vi "HB_SetTime.vi"(8 "error in (no error)":errorcluster, 10 "Time Stamp":timestamp, 11 "HBDeviceRef":T1) -> (0 "error IO":errorcluster, 3 "HBDeviceRef":T1)   [LabVIEW 2016]
uses:
  <vilib>/Rock Robotics/WPI/SerialPort/WPI_SerialPortRef.ctl
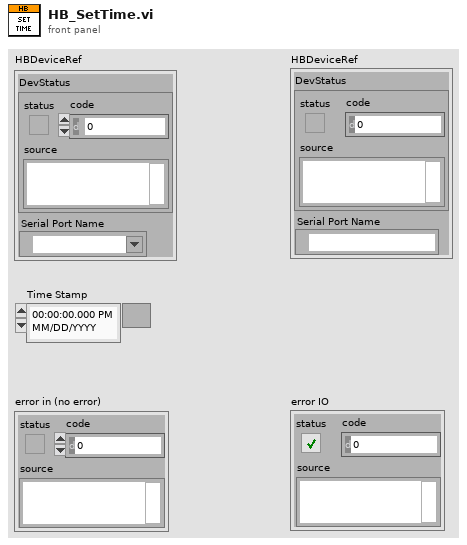
[diagram p1: front panel]
types:
  T1 = typedef "WPI_SerialPortRef.ctl" = cluster{"DevStatus":errorcluster, "Serial Port Name":refnum<visa-resource-name>}
  T2 = typedef "LVDateTimeRec.ctl" = cluster{"fractional second":dbl, "second":i32, "minute":i32, "hour":i32, "day of month":i32, "month":i32, "year":i32, "day of week":i32, "day of year":i32, "DST":i32}
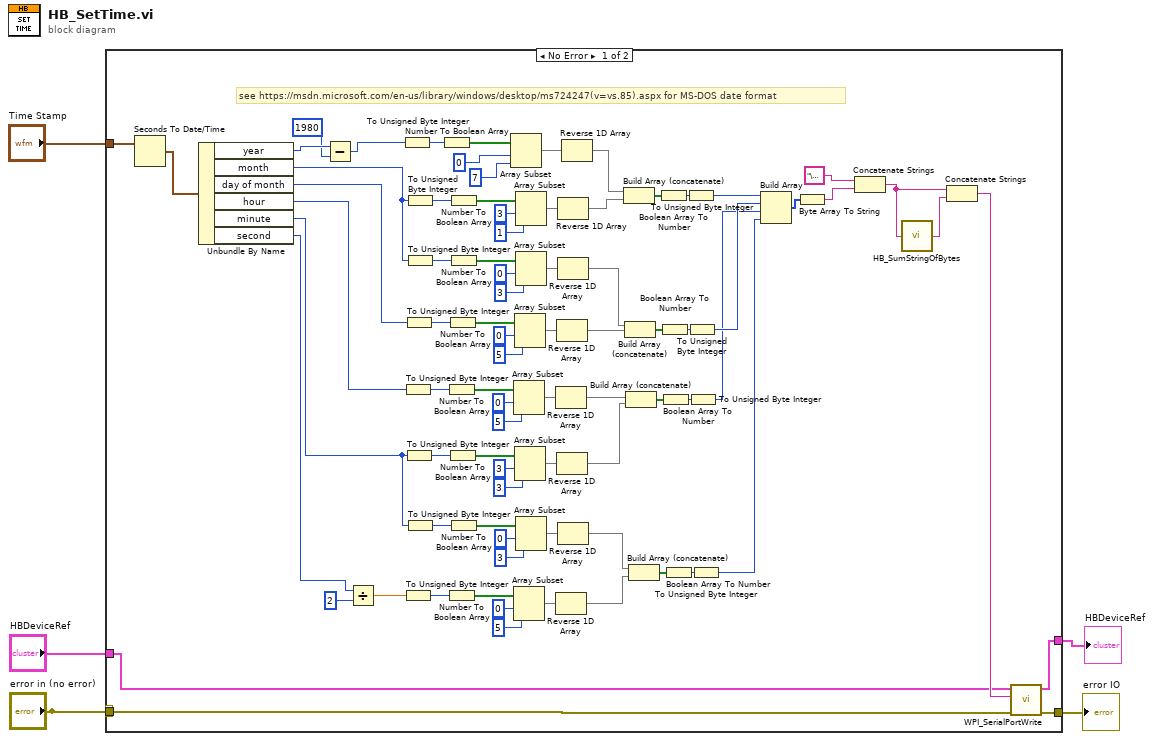
[diagram p0: block diagram]
diagram:
  n1 = case shown="No Error" "error in (no error)" {
    selector: "error in (no error)" -> [w9 w88]
    tunnel: "HBDeviceRef" -> [w6 w89]
    tunnel: "error in (no error)" -> [_ _]
    tunnel: [w7 w89] -> w2
    tunnel: [w8 w88] -> w3
    tunnel: "Time Stamp" -> [w66 _]
    frame No Error {
      # "see https://msdn.microsoft.com/en-us/library/windows/desktop/ms724247(v=vs.85).aspx for MS-DOS date format"
      n2 = Seconds To Date/Time(time stamp (now)=w66) -> (date time rec=w65:T2)  [unwired: 1 in]
      n3 = Unbundle By Name(w65) -> ("year"=w64:i32, "month"=w12:i32, "day of month"=w41:i32, "hour"=w40:i32, "minute"=w13:i32, "second"=w39:i32)
      n4 = Subtract(x=w64, y=1980) -> (x-y=w62:i32)
      n5 = Divide(x=w39, y=2) -> (x/y=w38:dbl)
      n6 = To Unsigned Byte Integer(number=w62) -> (unsigned 8bit integer=w78:u8)
      n7 = To Unsigned Byte Integer(number=w40) -> (unsigned 8bit integer=w56:u8)
      n8 = To Unsigned Byte Integer(number=w38) -> (unsigned 8bit integer=w46:u8)
      n9 = To Unsigned Byte Integer(number=w41) -> (unsigned 8bit integer=w61:u8)
      n10 = To Unsigned Byte Integer(number=w13) -> (unsigned 8bit integer=w51:u8)
      n11 = To Unsigned Byte Integer(number=w12) -> (unsigned 8bit integer=w83:u8)
      n12 = To Unsigned Byte Integer(number=w12) -> (unsigned 8bit integer=w30:u8)
      n13 = To Unsigned Byte Integer(number=w13) -> (unsigned 8bit integer=w21:u8)
      n14 = Number To Boolean Array(number=w78) -> (Boolean array=w77:bool[])
      n15 = Number To Boolean Array(number=w56) -> (Boolean array=w52:bool[])
      n16 = Number To Boolean Array(number=w46) -> (Boolean array=w42:bool[])
      n17 = Number To Boolean Array(number=w61) -> (Boolean array=w57:bool[])
      n18 = Number To Boolean Array(number=w51) -> (Boolean array=w47:bool[])
      n19 = Number To Boolean Array(number=w83) -> (Boolean array=w79:bool[])
      n20 = Number To Boolean Array(number=w30) -> (Boolean array=w26:bool[])
      n21 = Number To Boolean Array(number=w21) -> (Boolean array=w17:bool[])
      n22 = Array Subset(array=w77, index=0, length=7) -> (w68:bool[])
      n23 = Array Subset(array=w52, index=0, length=5) -> (w53:bool[])
      n24 = Array Subset(array=w42, index=0, length=5) -> (w43:bool[])
      n25 = Array Subset(array=w57, index=0, length=5) -> (w58:bool[])
      n26 = Array Subset(array=w47, index=3, length=3) -> (w48:bool[])
      n27 = Array Subset(array=w79, index=3, length=1) -> (w80:bool[])
      n28 = Array Subset(array=w26, index=0, length=3) -> (w27:bool[])
      n29 = Array Subset(array=w17, index=0, length=3) -> (w18:bool[])
      n30 = Reverse 1D Array(array=w53) -> (reversed array=w22:bool[])
      n31 = Reverse 1D Array(array=w43) -> (reversed array=w14:bool[])
      n32 = Reverse 1D Array(array=w58) -> (reversed array=w24:bool[])
      n33 = Reverse 1D Array(array=w48) -> (reversed array=w16:bool[])
      n34 = Reverse 1D Array(array=w80) -> (reversed array=w72:bool[])
      n35 = Reverse 1D Array(array=w27) -> (reversed array=w25:bool[])
      n36 = Reverse 1D Array(array=w18) -> (reversed array=w15:bool[])
      n37 = Reverse 1D Array(array=w68) -> (reversed array=w67:bool[])
      n38 = Build Array (concatenate)(w67, w72) -> (w71:bool[])
      n39 = Build Array (concatenate)(w25, w24) -> (w35:bool[])
      n40 = Build Array (concatenate)(w22, w16) -> (w33:bool[])
      n41 = Build Array (concatenate)(w15, w14) -> (w31:bool[])
      n42 = Boolean Array To Number(Boolean array=w71) -> (number=w75:u32)
      n43 = Boolean Array To Number(Boolean array=w35) -> (number=w36:u32)
      n44 = Boolean Array To Number(Boolean array=w33) -> (number=w34:u32)
      n45 = Boolean Array To Number(Boolean array=w31) -> (number=w32:u32)
      n46 = To Unsigned Byte Integer(number=w75) -> (unsigned 8bit integer=w74:u8)
      n47 = To Unsigned Byte Integer(number=w36) -> (unsigned 8bit integer=w23:u8)
      n48 = To Unsigned Byte Integer(number=w34) -> (unsigned 8bit integer=w11:u8)
      n49 = To Unsigned Byte Integer(number=w32) -> (unsigned 8bit integer=w10:u8)
      n50 = Build Array(w74, w23, w11, w10) -> (w73:u8[])
      n51 = Byte Array To String(unsigned byte array=w73) -> (string=w70:string)
      n52 = Concatenate Strings("\u0005", w70) -> (w85:string)
      n53 = call <vilib>:"HB_SumStringOfBytes.vi"("String Of Bytes"=w85) -> ("Sum as String"=w84:string)
      n54 = Concatenate Strings(w85, w84) -> (w86:string)
      n55 = call <vilib>:"WPI_SerialPortWrite.vi"("error in (no error)"=w9, "Buffer"=w86, "SerialPortRef"=w6) -> ("error out"=w8:errorcluster, "SerialPortRef"=w7:T1)  [unwired: 6 in, 1 out]
    }
    frame Error {
    }
  }
  "HBDeviceRef" <- w2
  "error IO" <- w3
